vi "SubVI - Get Connected Indicators.vi"(8 "error in (no error)":errorcluster, 11 "SubVI in":refnum<vi>) -> (0 "error out":errorcluster, 3 "Array 2":refnum<vi>[](array[refnum]))   [LabVIEW 2017, in "csmHelper-SubVI.lvlib"]
uses:
  csmHelper-SubVI.lvlib
  Terminals/csmHelper-Terminals.lvlib
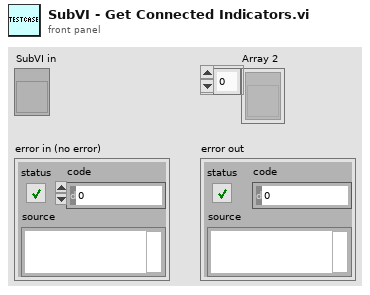
[diagram p1: front panel]
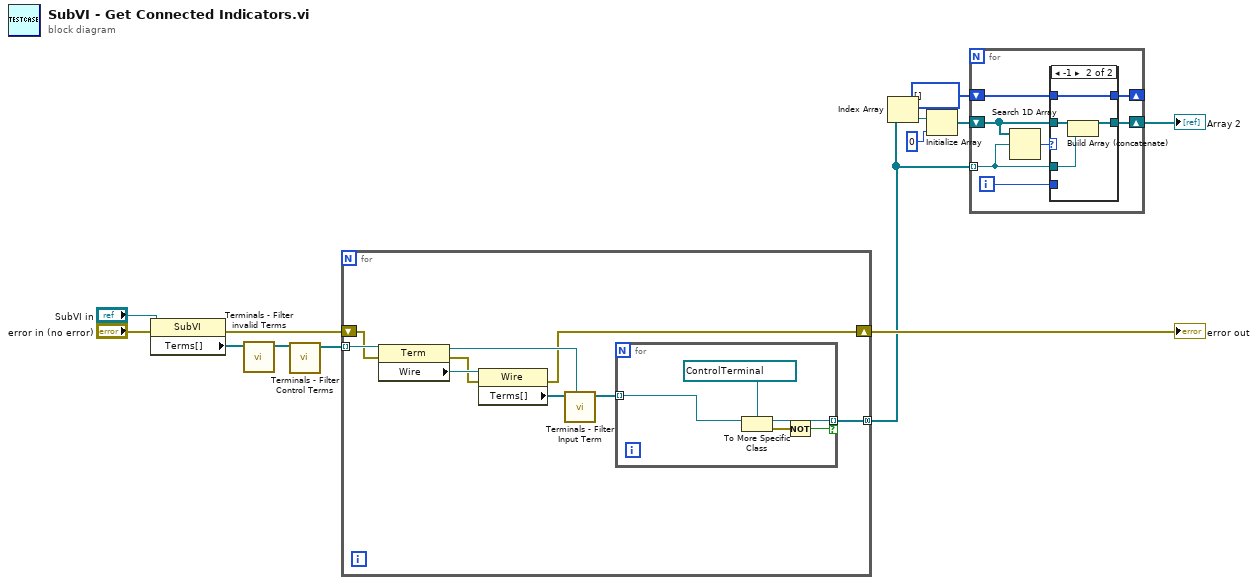
[diagram p0: block diagram]
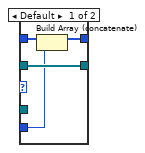
[diagram p2: hidden frame]
diagram:
  n1 = property on="Property Node" class="SubVI"(reference="SubVI in", error in="error in (no error)") -> (error out=w7:errorcluster, "Terms[]"=w5:refnum<vi>[])  [unwired: 1 out]
  n2 = call "Terminals - Filter invalid Terms.vi"("Terms[]"=w5) -> ("Terms[] out"=w1:refnum<vi>[])  [unwired: 10 in]
  n3 = call "Terminals - Filter Control Terms.vi"("Terms[]"=w1) -> ("Terms[] out"=w6:refnum<vi>[])  [unwired: 10 in]
  n4 = for {
    tunnel: w6 -> [w22] mode=indexing
    shift-right: [w15] -> w13
    shift-left: w7 -> [w16]
    tunnel: [w14] -> w12 mode=concatenating
    n5 = property class="Term"(reference=w22, error in=w16) -> (reference out=w19:refnum<vi>, error out=w17:errorcluster, "Wire"=w21:refnum<vi>)
    n6 = property class="Wire"(reference=w21, error in=w17) -> (error out=w15:errorcluster, "Terms[]"=w20:refnum<vi>[])  [unwired: 1 out]
    n7 = call "Terminals - Filter Input Term.vi"("InnerTerminal in"=w19, "Wire.Terms[] in"=w20) -> ("Wire.Terms[] out"=w18:refnum<vi>[])  [unwired: 9 in]
    n8 = for {
      tunnel: w18 -> [w23] mode=indexing
      tunnel: [w26] -> w14 mode=indexing if=w24
      n9 = To More Specific Class(target class=refnum<vi> refnum ("reference out"), reference=w23) -> (specific class reference=w26:refnum<vi>, error out=w25:errorcluster)  [unwired: 1 in]
      n10 = Not(x=w25) -> (.not. x?=w24:bool)
    }
  }
  "error out" <- w13
  n11 = Index Array(array=w12) -> (element=w9:refnum<vi>)  [unwired: 1 in]
  n12 = Initialize Array(w9, 0 ("Dimension Size")) -> (w10:refnum<vi>[])
  n13 = for {
    tunnel: w12 -> [w33] mode=indexing
    shift-right: [w32] -> w2
    shift-left: w10 -> [w31]
    shift-right: [w29] -> _
    shift-left: i32[] [] -> [w28]
    i -> [w30]
    n14 = Search 1D Array(1D array=w31, element=w33) -> (index of element=w34:i32)  [unwired: 1 in]
    n15 = case shown="-1" w34 {
      tunnel: w33 -> [_ w42]
      tunnel: [w38 w40] -> w32
      tunnel: w31 -> [w38 w41]
      tunnel: w30 -> [w35 _]
      tunnel: [w36 w39] -> w29
      tunnel: w28 -> [w37 w39]
      frame Default {
        n16 = Build Array (concatenate)(w37, w35) -> (w36:i32[])
      }
      frame -1 {
        n17 = Build Array (concatenate)(w41, w42) -> (w40:refnum<vi>[])
      }
    }
  }
  "Array 2" <- w2
